vi "sync_1.vi"(4 "error in":errorcluster, 5 "dpd":dbl=3000.0, 6 "group name":string, 7 "tdms file out":refnum<k34>) -> (0 "error out":errorcluster, 1 "Waveform":waveform(dbl), 2 "other_chans":string[](array[string]), 3 "tdms file out 2":refnum<k34>)   [LabVIEW 2010]
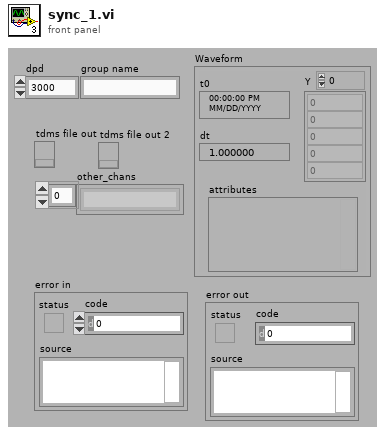
[diagram p1: front panel]
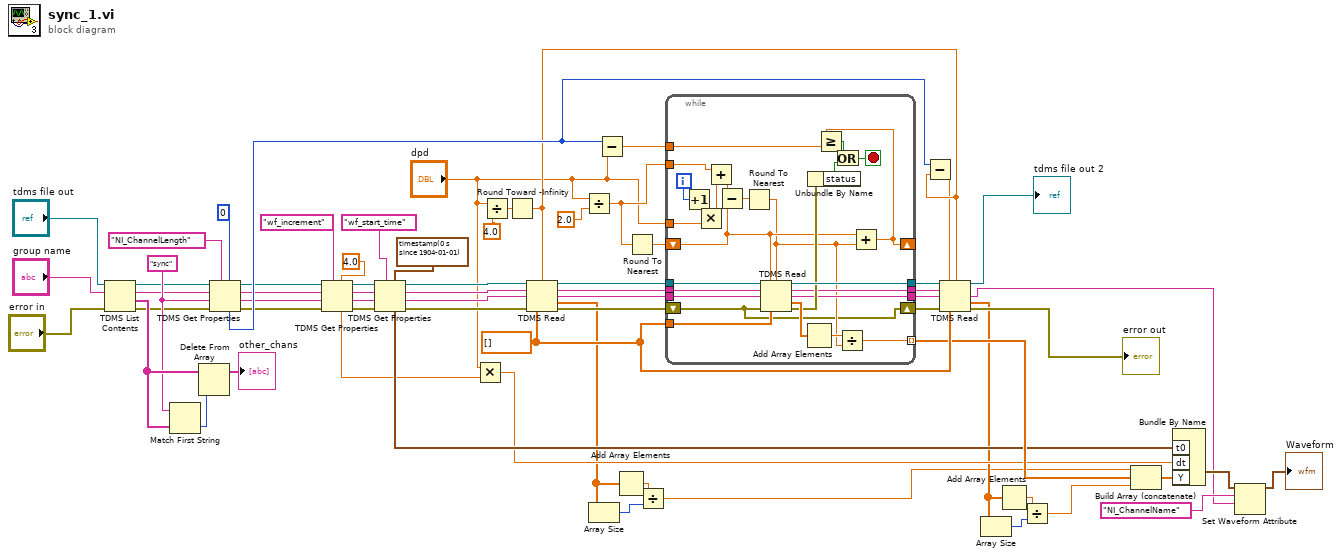
[diagram p0: block diagram]
diagram:
  w7 = "sync" ("channel name")
  w50 = dbl[] []
  n1 = TDMS List Contents(4:"error in", 6:"group name", 7:"tdms file out") -> (0:w3:errorcluster, 1:w8:string[], 2:w5:string, 3:w4:refnum<k34>)
  n2 = Match First String(2:w8, 3:w7) -> (0:w12:i32)  [unwired: 1 out]
  n3 = Delete From Array(array=w8, index=w12) -> (array with subset deleted=→"other_chans":string[])  [unwired: 1 in, 1 out]
  n4 = TDMS Get Properties(5:0, 7:"NI_ChannelLength", 8:w3, 9:w7, 10:w5, 11:w4) -> (0:w21:errorcluster, 1:w20:string, 2:w19:string, 3:w18:refnum<k34>, 4:w65:i32)  [unwired: 1 out]
  n5 = TDMS Get Properties(5:4.0 ("count (-1: all)"), 7:"wf_increment", 8:w21, 9:w20, 10:w19, 11:w18) -> (0:w37:errorcluster, 1:w38:string, 2:w39:string, 3:w40:refnum<k34>, 4:w27:dbl)  [unwired: 1 out]
  n6 = TDMS Get Properties(5:timestamp(0 s since 1904-01-01), 7:"wf_start_time", 8:w37, 9:w38, 10:w39, 11:w40) -> (0:w36:errorcluster, 1:w33:string, 2:w34:string, 3:w35:refnum<k34>, 4:w29:timestamp)  [unwired: 1 out]
  n7 = Multiply(x="dpd", y=w27) -> (x*y=w26:dbl)
  n8 = Divide(x="dpd", y=4.0 ("count (-1: all)")) -> (x/y=w47:dbl)
  n9 = Round Toward -Infinity(1:w47) -> (0:w52:dbl)
  n10 = TDMS Read(0:w35, 2:w52, 5:w34, 7:w33, 11:w36, 12:w50) -> (4:w45:refnum<k34>, 6:w55:string, 8:w56:string, 10:w14:dbl[], 15:w53:errorcluster)  [unwired: 1 in, 1 out]
  n11 = Divide(x="dpd", y=2.0 ("count (-1: all)")) -> (x/y=w62:dbl)
  n12 = Array Size(array=w14) -> (size(s)=w13:i32)
  n13 = Subtract(x=w65, y="dpd") -> (x-y=w59:dbl)
  n14 = Add Array Elements(numeric array=w14) -> (sum=w48:dbl)
  n15 = Round To Nearest(number=w62) -> (nearest integer value=w61:dbl)
  n16 = Divide(x=w48, y=w13) -> (x/y=w1:dbl)
  n17 = while {
    tunnel: w45 -> [w92]
    tunnel: [w91] -> w41
    tunnel: w55 -> [w90]
    tunnel: w56 -> [w89]
    tunnel: w50 -> [w88]
    tunnel: [w67] -> w44 mode=indexing
    shift-right: [w68] -> w54
    shift-left: w53 -> [w68]
    tunnel: [w81] -> w57
    tunnel: [w80] -> w58
    shift-right: [w79] -> _
    shift-left: w61 -> [w71]
    tunnel: w59 -> [w78]
    tunnel: "dpd" -> [w74]
    tunnel: w62 -> [w73]
    i -> [w75]
    stop <- w83 stop-if-true
    n18 = Increment(x=w75) -> (x+1=w77:i32)
    n19 = Multiply(x=w77, y=w74) -> (x*y=w76:dbl)
    n20 = Add(x=w73, y=w76) -> (x+y=w72:dbl)
    n21 = Subtract(x=w72, y=w71) -> (x-y=w70:dbl)
    n22 = Round To Nearest(number=w70) -> (nearest integer value=w69:dbl)
    n23 = TDMS Read(0:w92, 1:w71, 2:w69, 5:w90, 7:w89, 11:w68, 12:w88) -> (4:w91:refnum<k34>, 6:w81:string, 8:w80:string, 10:w87:dbl[], 15:w85:errorcluster)  [unwired: 1 out]
    n24 = Add Array Elements(numeric array=w87) -> (sum=w86:dbl)
    n25 = Unbundle By Name(w85) -> ("status"=w84:bool)
    n26 = Divide(x=w86, y=w69) -> (x/y=w67:dbl)
    n27 = Add(x=w71, y=w69) -> (x+y=w79:dbl)
    n28 = Greater Or Equal?(x=w79, y=w78) -> (x >= y?=w82:bool)
    n29 = Or(x=w82, y=w84) -> (x .or. y?=w83:bool)
  }
  n30 = Subtract(x=w65, y=w52) -> (x-y=w51:dbl)
  n31 = TDMS Read(0:w41, 1:w51, 2:w52, 5:w57, 7:w58, 11:w54, 12:w50) -> (4:→"tdms file out 2":refnum<k34>, 8:w17:string, 10:w16:dbl[], 15:→"error out":errorcluster)  [unwired: 2 out]
  n32 = Array Size(array=w16) -> (size(s)=w15:i32)
  n33 = Add Array Elements(numeric array=w16) -> (sum=w49:dbl)
  n34 = Divide(x=w49, y=w15) -> (x/y=w2:dbl)
  n35 = Build Array (concatenate)(w1, w44, w2) -> (w42:dbl[])
  n36 = Bundle By Name("t0"=w29, "dt"=w26, "Y"=w42) -> (w24:waveform(dbl))  [unwired: 1 in]
  n37 = Set Waveform Attribute(5:w17, 6:"NI_ChannelName", 7:w24) -> (3:→"Waveform":waveform(dbl))  [unwired: 1 in, 2 out]
